vi "Multiple Instances.vi"() -> ()   [LabVIEW 2020]
uses:
  C:/Users/Simon/Documents/GitHub/LV-WebView2/Source/Libs/Microsoft.Web.WebView2.WinForms.dll
  Libs/Microsoft.Web.WebView2.WinForms.dll
  Webview2 Lib/WebView2 Control Object/WebView2 Control.lvclass
panel:
  in  "WebView2":refnum<k24>(container)
  in  "WebView2 2":refnum<k24>(container)
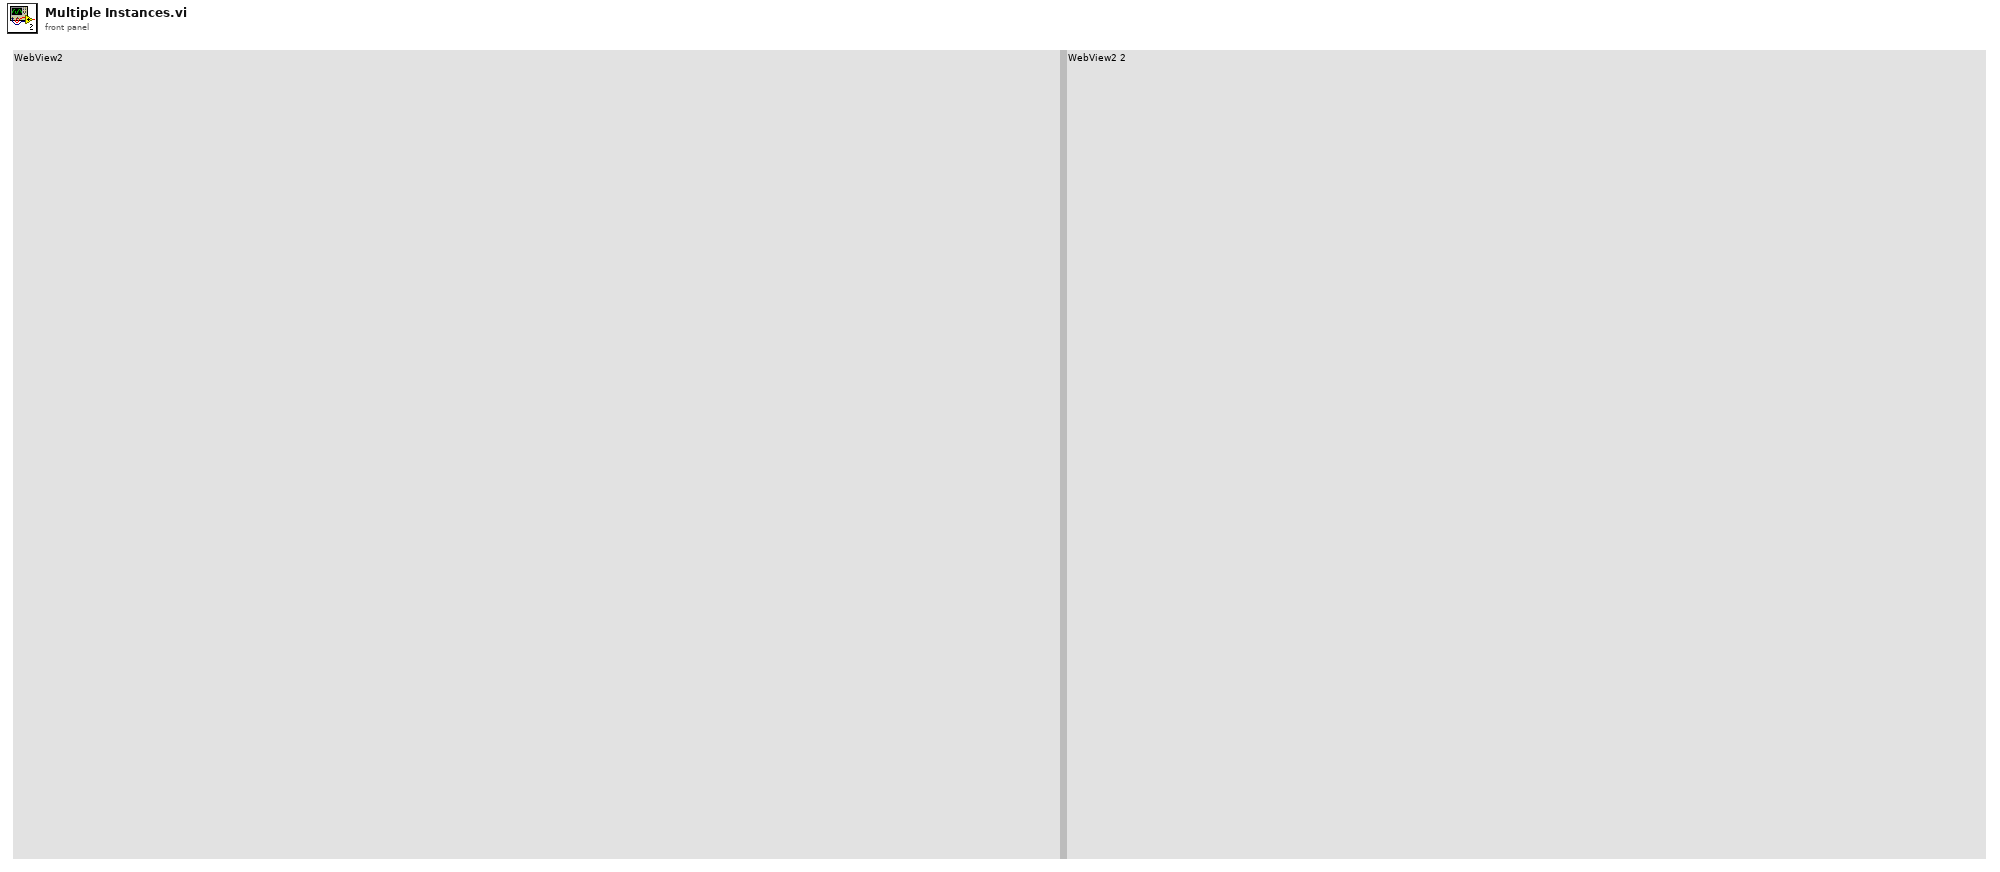
[diagram p1: front panel]
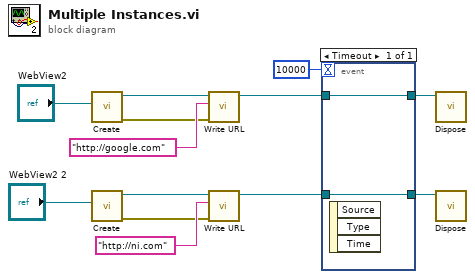
[diagram p0: block diagram]
diagram:
  n1 = call "Create.vi"("WebView2 Control"="WebView2") -> ("error out"=w1:errorcluster, "WebView2 Control out"=w12:refnum<class "WebView2 Control.lvclass">)  [unwired: 9 in]
  n2 = call "Create.vi"("WebView2 Control"="WebView2 2") -> ("error out"=w2:errorcluster, "WebView2 Control out"=w10:refnum<class "WebView2 Control.lvclass">)  [unwired: 9 in]
  n3 = call "Write URL.vi"("error in (no error)"=w1, "uri"="http://google.com" ("WebView2 Control 2"), "WebView2 Control in"=w12) -> ("WebView2 Control out"=w5:refnum<class "WebView2 Control.lvclass">)  [unwired: 7 in, 1 out]
  n4 = call "Write URL.vi"("error in (no error)"=w2, "uri"="http://ni.com" ("WebView2 Control"), "WebView2 Control in"=w10) -> ("WebView2 Control out"=w6:refnum<class "WebView2 Control.lvclass">)  [unwired: 7 in, 1 out]
  n5 = event shown="[0] Timeout" {
    selector: _ -> [_]
    dyn-events: _ -> [_]
    timeout: 10000 -> [_]
    tunnel: [w15] -> w8
    tunnel: w5 -> [w15]
    tunnel: [w14] -> w7
    tunnel: w6 -> [w14]
    event Timeout {
      n6 = event-data() -> ()  [unwired: 1 in, 3 out]
    }
  }
  n7 = call "Dispose.vi"("WebView2 Control in"=w8) -> ()  [unwired: 10 in, 1 out]
  n8 = call "Dispose.vi"("WebView2 Control in"=w7) -> ()  [unwired: 10 in, 1 out]
